vi "ConfigureHWSynced.vi"(0 "object in":refnum<class "Hamamatsu.lvclass">, 2 "FramesPerAquisionCycle":i32, 3 "CameraBufferSize":i32, 5 "error in (no error)":errorcluster) -> (14 "object out":refnum<class "Hamamatsu.lvclass">, 19 "error out":errorcluster)   [LabVIEW 2019, in "Hamamatsu.lvclass"]
uses:
  Hamamatsu.lvclass
  Hamamatsu.lvclass/Hamamatsu.ctl
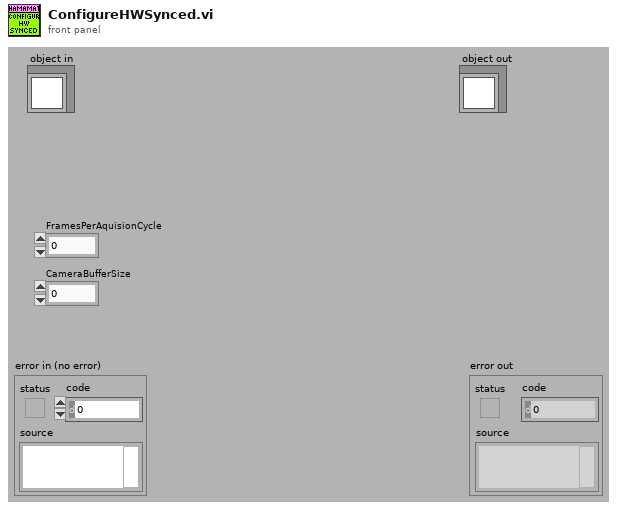
[diagram p1: front panel]
types:
  T1 = typedef "IMAQ Image.ctl" = refnum<image>
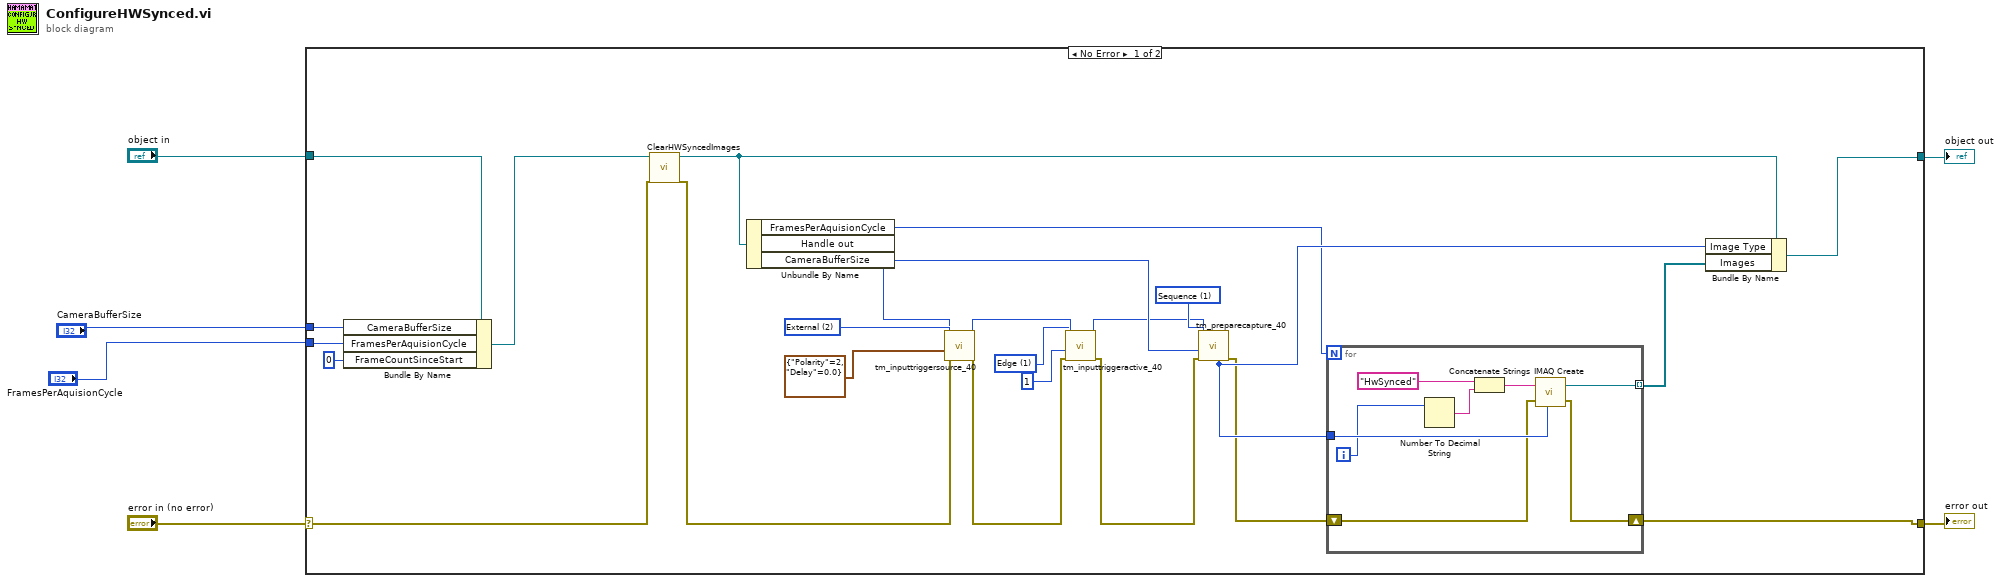
[diagram p0: block diagram]
diagram:
  n1 = case shown="No Error" "error in (no error)" {
    selector: "error in (no error)" -> [w14 w41]
    tunnel: [w26 w41] -> w5
    tunnel: [w27 w40] -> w3
    tunnel: "object in" -> [w9 w40]
    tunnel: "CameraBufferSize" -> [w8 _]
    tunnel: "FramesPerAquisionCycle" -> [w11 _]
    frame No Error {
      w20 = 1 items=["Edge"=1, "Level"=2, "Sync Readout"=3, "Point"=4] ("Active")
      w25 = 2 items=["Internal"=1, "External"=2, "Software"=3, "Master Pulse"=4] ("Source")
      w31 = 1 items=["Snap", "Sequence"] ("Capture mode")
      n2 = Bundle By Name(cluster=w9, "CameraBufferSize"=w8, "FramesPerAquisionCycle"=w11, "FrameCountSinceStart"=0) -> (w10:refnum<class "Hamamatsu.lvclass">)
      n3 = call-dynamic "ClearHWSyncedImages.vi"("object in"=w10, "error in (no error)"=w14) -> ("object out"=w15:refnum<class "Hamamatsu.lvclass">, "error out"=w13:errorcluster)  [unwired: 16 in]
      n4 = Unbundle By Name(w15) -> ("FramesPerAquisionCycle"=w12:i32, "Handle out"=w24:u32, "CameraBufferSize"=w28:i32)
      n5 = call <userlib>:"tm_inputtriggersource_40.vi"("error in (no error)"=w13, "External Options"=cluster{"Polarity":i32, "Delay":dbl} {"Polarity"=2, "Delay"=0.0}, "Source"=w25, "Handle in"=w24) -> ("error out"=w18:errorcluster, "Handle out"=w22:u32)  [unwired: 6 in]
      n6 = call <userlib>:"tm_inputtriggeractive_40.vi"("error in (no error)"=w18, "Times"=1, "Active"=w20, "Handle in"=w22) -> ("error out"=w17:errorcluster, "Handle out"=w21:u32)  [unwired: 6 in]
      n7 = call <userlib>:"tm_preparecapture_40.vi"("error in (no error)"=w17, "Frames"=w28, "Capture mode"=w31, "Handle in"=w21) -> ("error out"=w29:errorcluster, "Image type"=w30:u32)  [unwired: 4 in, 2 out]
      n8 = for {
        N: w12 -> [_]
        tunnel: w30 -> [w38]
        shift-right: [w36] -> w26
        shift-left: w29 -> [w37]
        tunnel: [w35] -> w16 mode=indexing
        i -> [w34]
        n9 = Number To Decimal String(number=w34) -> (decimal integer string=w32:string)  [unwired: 1 in]
        n10 = Concatenate Strings("HwSynced" ("Image Name"), w32) -> (w33:string)
        n11 = call "IMAQ Create"("Image Name"=w33, "Image Type"=w38, "error in (no error)"=w37) -> ("New Image"=w35:T1, "error out"=w36:errorcluster)  [unwired: 2 in]
      }
      n12 = Bundle By Name(cluster=w15, "Image Type"=w30, "Images"=w16) -> (w27:refnum<class "Hamamatsu.lvclass">)
    }
    frame Error {
    }
  }
  "error out" <- w5
  "object out" <- w3
